vi "SW_Gen_2D_Histogram.vi"(7 "Picture reference in":refnum<vi>, 8 "Pixels per mm":dbl, 9 "Y coord array":dbl[](array[numeric]), 10 "X coord array":dbl[](array[numeric]), 11 "Bounds":T1) -> (2 "24-bit pixmap":u32[][](array[numeric]), 3 "Picture":picture)   [LabVIEW 2016]
uses:
  <vilib>/Utility/miscctls.llb/LVBoundsTypeDef.ctl
  <vilib>/Heliosphere Research LLC/Advanced Plotting Toolkit/api_core/NewPlotType.ctl
  <vilib>/Heliosphere Research LLC/Advanced Plotting Toolkit/api_plotting/Histogram2DRange.ctl
  <vilib>/Heliosphere Research LLC/Advanced Plotting Toolkit/api_core/NewPlotProperties.ctl
  <vilib>/Heliosphere Research LLC/Advanced Plotting Toolkit/typedefs/PlotColor.ctl
  <vilib>/Heliosphere Research LLC/Advanced Plotting Toolkit/api_plotting/Histogram2DProperties.ctl
  <vilib>/Heliosphere Research LLC/Advanced Plotting Toolkit/properties/Colormap.ctl
  <vilib>/Heliosphere Research LLC/Advanced Plotting Toolkit/properties/Colormap_Map.ctl
  <vilib>/Heliosphere Research LLC/Advanced Plotting Toolkit/properties/Colormap_Scaling.ctl
  <vilib>/Heliosphere Research LLC/Advanced Plotting Toolkit/properties/Display.ctl
  <vilib>/Heliosphere Research LLC/Advanced Plotting Toolkit/api_plotting/Histogram2D_Automatic.vi
  <vilib>/Heliosphere Research LLC/Advanced Plotting Toolkit/Advanced Plotting Toolkit.lvlib
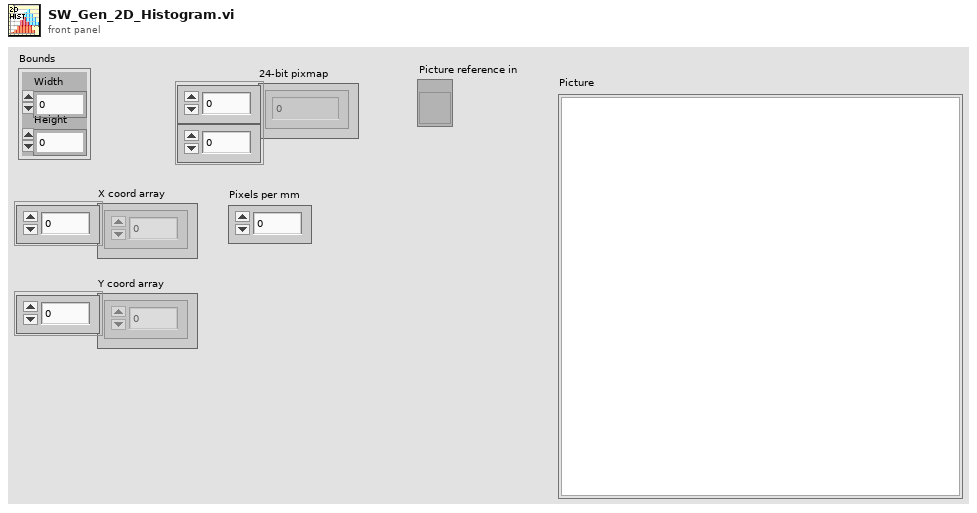
[diagram p1: front panel]
types:
  T1 = typedef "LVBoundsTypeDef.ctl" = cluster{"Width":u32, "Height":u32}
  T2 = typedef "Advanced Plotting Toolkit.lvlib/Histogram2DProperties.ctl" = cluster{"Normalize":bool, "Colormap":T3, "Display":T6}
  T3 = typedef "Advanced Plotting Toolkit.lvlib/Colormap.ctl" = cluster{"Map":T4, "Value Min":dbl, "Value Max":dbl, "Scaling":T5, "Reverse":bool}
  T4 = typedef "Advanced Plotting Toolkit.lvlib/Colormap_Map.ctl" = enum16{"Automatic", "Rainbow", "Hot and Cold", "White-Black", "White-Blue", "White-Green", "White-Red", "Fire", "Water", "Earth", "Air", "Pastel", "Banded", "Stepped"}
  T5 = typedef "Advanced Plotting Toolkit.lvlib/Colormap_Scaling.ctl" = enum16{"Default"}
  T6 = typedef "Advanced Plotting Toolkit.lvlib/Display.ctl" = cluster{"Alpha":dbl, "Z Order":dbl}
  T7 = typedef "Advanced Plotting Toolkit.lvlib/NewPlotProperties.ctl" = cluster{"Background Color":T8, "Axis Background":T8, "Left Margin":dbl, "Right Margin":dbl, "Bottom Margin":dbl, "Top Margin":dbl, "Aspect Ratio":dbl}
  T8 = typedef "Advanced Plotting Toolkit.lvlib/PlotColor.ctl" = u32
  T9 = typedef "Advanced Plotting Toolkit.lvlib/Histogram2DRange.ctl" = cluster{"X Min":dbl, "X Max":dbl, "Y Min":dbl, "Y Max":dbl}
  T10 = typedef "Advanced Plotting Toolkit.lvlib/NewPlotType.ctl" = enum16{"Rectangular Axes", "Polar Axes"}
  T11 = typedef "Advanced Plotting Toolkit.lvlib/PlotID.ctl" = i32
  T12 = typedef "imagedata.ctl" = cluster{"image type":i32, "image depth":i32, "image":u8[], "mask":u8[], "colors":u32[], "Rectangle":cluster{"left":i16, "top":i16, "right":i16, "bottom":i16}}
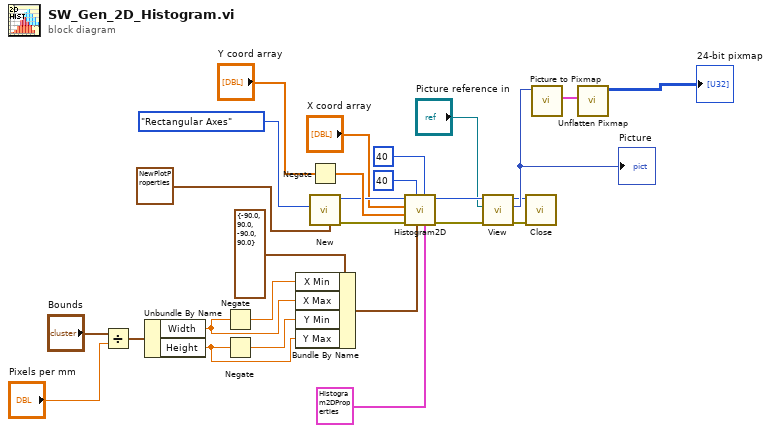
[diagram p0: block diagram]
diagram:
  n1 = Divide(x="Bounds", y="Pixels per mm") -> (x/y=w23:cluster{"Width":dbl, "Height":dbl})
  n2 = Unbundle By Name(w23) -> ("Width"=w24:dbl, "Height"=w25:dbl)
  n3 = Negate(x=w24) -> (-x=w26:dbl)
  n4 = Negate(x=w25) -> (-x=w27:dbl)
  n5 = Bundle By Name(cluster=T9 {"X Min"=-90.0, "X Max"=90.0, "Y Min"=-90.0, "Y Max"=90.0} ("Data Range"), "X Min"=w26, "X Max"=w24, "Y Min"=w27, "Y Max"=w25) -> (w22:T9)
  n6 = Negate(x="Y coord array") -> (-x=w15:dbl[])
  n7 = call <vilib>:"New.vi"("Properties"=T7 {"Background Color"=2147483647, "Axis Background"=2147483647, "Left Margin"=0.0, "Right Margin"=0.0, "Bottom Margin"=0.0, "Top Margin"=0.0, "Aspect Ratio"=1.0} ("Plot properties"), "Plot Type"=NewPlotType."Rectangular Axes") -> ("error out"=w8:errorcluster, "Plot ID"=w6:T11)  [unwired: 8 in]
  n8 = call-poly <vilib>:"Histogram2D.vi"("Properties"=T2 {"Normalize"=TRUE, "Colormap"={"Map"=enum."Rainbow", "Value Min"=nan, "Value Max"=nan, "Scaling"=enum."Default", "Reverse"=FALSE}, "Display"={"Alpha"=1.0, "Z Order"=nan}} ("Histogram properties"), "Y Bins"=40, "Data Range"=w22, "X Bins"=40, "error in (no error)"=w8, "Y Data"=w15, "X Data"="X coord array", "Plot ID"=w6) -> ("error out"=w9:errorcluster, "Plot ID Out"=w18:T11)  [unwired: 2 in]
  n9 = call <vilib>:"View.vi"("error in (no error)"=w9, "Ref for Sizing"="Picture reference in", "Plot ID"=w18) -> ("error out"=w12:errorcluster, "Picture"=w19:picture, "Plot ID Out"=w11:T11)  [unwired: 6 in]
  "Picture" <- w19
  n10 = call <vilib>:"Close.vi"("error in (no error)"=w12, "Plot ID"=w11) -> ()  [unwired: 9 in, 1 out]
  n11 = call <vilib>:"Picture to Pixmap.vi"("picture"=w19) -> ("image data"=w20:T12)  [unwired: 9 in, 1 out]
  n12 = call <vilib>:"Unflatten Pixmap.vi"("image data"=w20) -> ("24-bit pixmap"=→"24-bit pixmap":u32[][])  [unwired: 4 in, 6 out]
